vi "Tag Expr Eval.vi"(8 "error in (no error)":errorcluster, 11 "Tag Expr in":refnum<class "Tag Expr.lvclass">) -> (0 "error out":errorcluster, 1 "Boolean Result":bool, 2 "Result":dbl format="%#_13g", 3 "Tag Expr out":refnum<class "Tag Expr.lvclass">)   [LabVIEW 2020, in "Tag Expr.lvclass"]
doc: "This VI looks up current Tag values then evaluates the expression.\n\nThe Boolean result is true if the numeric result is not equal to zero or NaN."
uses:
  Tag Expr.lvclass
  C:/Program Files (x86)/National Instruments/LabVIEW 2020/vi.lib/LAVA/muParser/mupExpr/mupExpr.lvclass
  Tag Expr.lvclass/Tag Expr.ctl
  Tag/Tag.lvclass/Tag.ctl
  <vilib>/LAVA/muParser/mupExpr/mupExpr.lvclass/mupExpr.ctl
  <vilib>/LAVA/muParser/mupExpr/Eval_SglRes.vi
  <vilib>/LAVA/muParser/mupLib/mupEval.vi
  Core/Get Tag Value_ByRef.vi
  <vilib>/LAVA/muParser/mupExpr/Set_Var_Value.vi
  <vilib>/LAVA/muParser/mupExpr/Set_MultiVar_Value.vi
  <vilib>/LAVA/muParser/mupLib/mupCheckError.vi
  Tag/Read Value.vi
  Tag/Read Timestamp.vi
  <vilib>/LAVA/muParser/mupExpr/SetVarVal.vi
  <vilib>/LAVA/muParser/mupLib/mupSetVarValue.vi
  <vilib>/Utility/error.llb/Error Cluster From Error Code.vi
  <vilib>/LAVA/muParser/mupExpr/mupExpr.lvclass
  C:/Users/leonidas/Documents/GitHub/tag-engine/Tag Expr/Tag Expr.lvclass
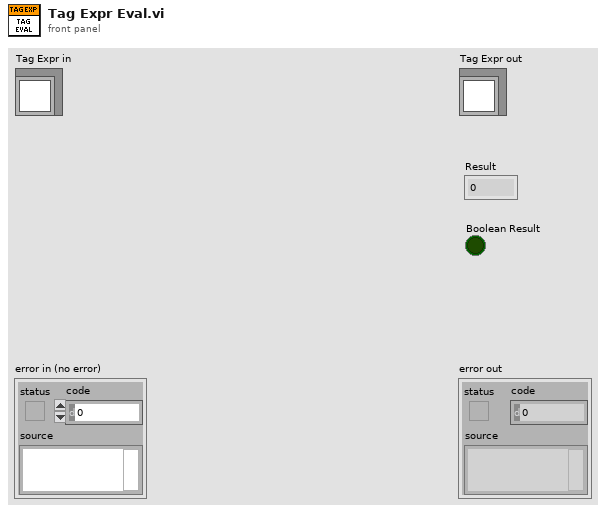
[diagram p1: front panel]
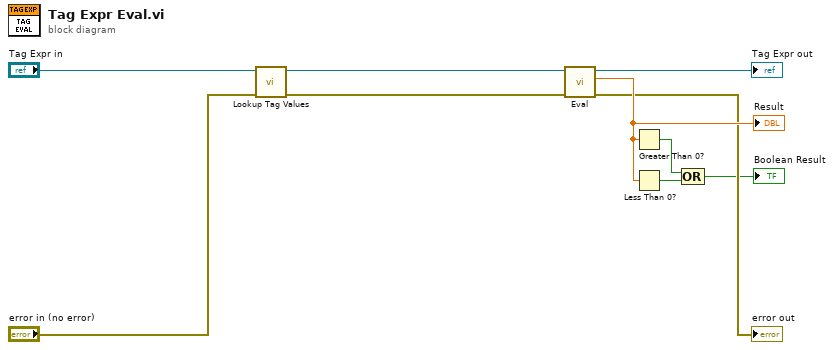
[diagram p0: block diagram]
diagram:
  n1 = call "Lookup Tag Values.vi"("error in (no error)"="error in (no error)", "Tag Expr in"="Tag Expr in") -> ("error out"=w2:errorcluster, "Tag Expr out"=w5:refnum<class "Tag Expr.lvclass">)  [unwired: 8 in]
  n2 = call-poly <vilib>:"Eval.vi"("error in (no error)"=w2, "muExpr in"=w5) -> ("error out"=→"error out":errorcluster, "Result"=w7:dbl, "muExpr out"=→"Tag Expr out":refnum<class "Tag Expr.lvclass">)  [unwired: 7 in]
  "Result" <- w7
  n3 = Greater Than 0?(x=w7) -> (x > 0?=w9:bool)
  n4 = Less Than 0?(x=w7) -> (x < 0?=w8:bool)
  n5 = Compound Arithmetic op=OR(w9, w8) -> (→"Boolean Result":bool)
